vi "Model - Set Elevator State.vi"(8 "error in (no error)":errorcluster, 10 "Elevator State":T1(ring), 11 "View Model":T2) -> (0 "error out":errorcluster, 3 "View Model":T2)   [LabVIEW 2017]
doc: "Using for Set current Elevator State"
uses:
  Controls/View Model.ctl
  Error Handler/Controls/Error Model.ctl
  Error Handler/Controls/Error Type.ctl
  Controls/Shared Model.ctl
  Elevator Controller/Controls/Elevator Model.ctl
  Elevator Controller/Controls/Controller Overhead.ctl
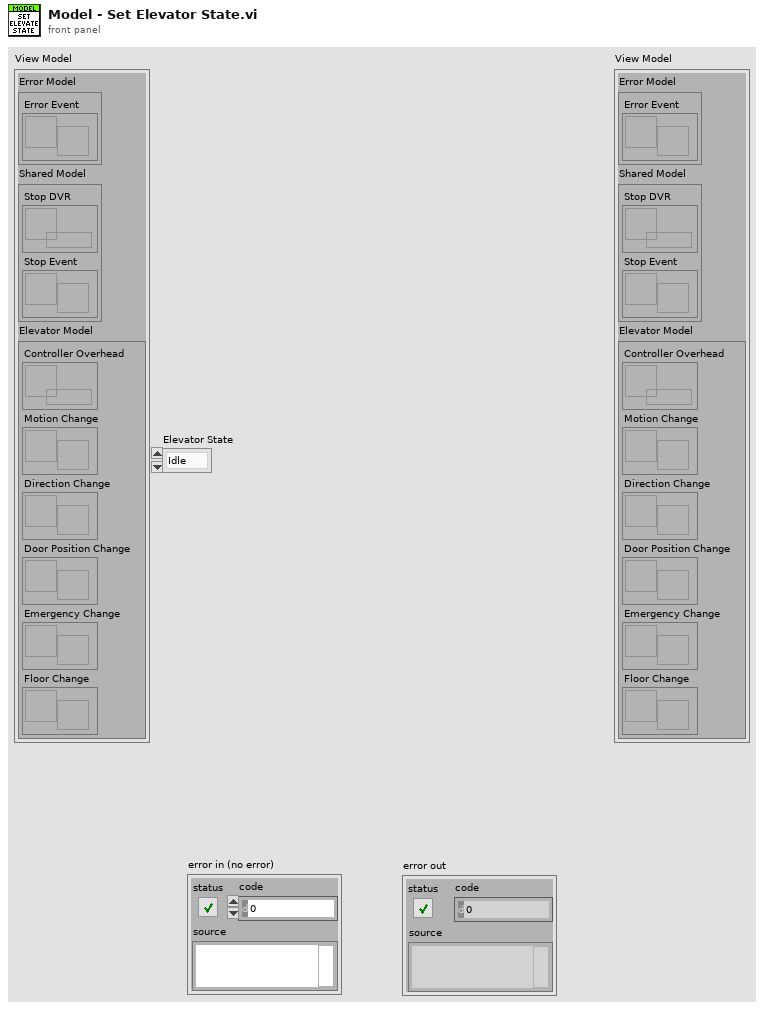
[diagram p1: front panel]
types:
  T1 = enum16{"Idle", "Open Doors", "Close Doors", "Travel", "Emergency"}
  T2 = typedef "View Model.ctl" = cluster{"Error Model":T3, "Shared Model":T4, "Elevator Model":T5}
  T3 = typedef "Error Model.ctl" = cluster{"Error Event":refnum<user-event>}
  T4 = typedef "Shared Model.ctl" = cluster{"Stop DVR":refnum<data-value>, "Stop Event":refnum<user-event>}
  T5 = typedef "Elevator Model.ctl" = cluster{"Controller Overhead":refnum<data-value>, "Motion Change":refnum<user-event>, "Direction Change":refnum<user-event>, "Door Position Change":refnum<user-event>, "Emergency Change":refnum<user-event>, "Floor Change":refnum<user-event>}
  T6 = typedef "Controller Overhead.ctl" = cluster{"In Motion?":bool, "Direction":bool, "Door Movement":bool, "Elevator State":enum16{"Idle", "Open Doors", "Close Doors", "Travel", "Emergency"}, "Next Elevator State":enum16{"Idle", "Open Doors", "Close Doors", "Travel", "Emergency"}, "Timer":dbl, "Elapsed Time":dbl, "Door Position":bool}
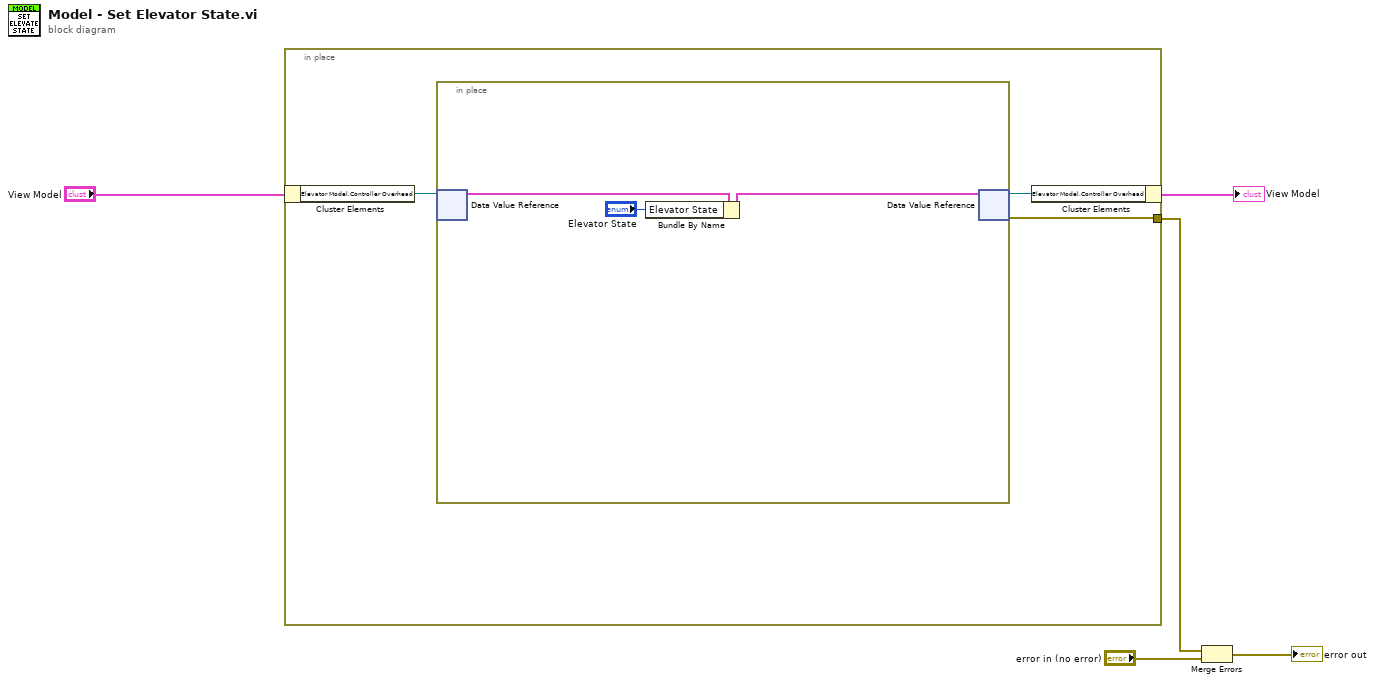
[diagram p0: block diagram]
diagram:
  n1 = in-place {
    in-place-border: [w7] -> w3
    n2 = in-place-cluster #1("View Model") -> ("Elevator Model.Controller Overhead"=w8:refnum<data-value>)
    n3 = in-place {
      n4 = in-place-dvr #2(w8) -> (w11:T6)  [unwired: 1 out]
      n5 = Bundle By Name(cluster=w11, "Elevator State"="Elevator State") -> (w10:T6)
      n6 = in-place-dvr #2(w10) -> (w6:refnum<data-value>, w7:errorcluster)
    }
    n7 = in-place-cluster #1("Elevator Model.Controller Overhead"=w6) -> (→"View Model":T2)
  }
  n8 = Merge Errors(w3, "error in (no error)") -> (→"error out":errorcluster)
